vi "Target Main.vi"() -> ()   [LabVIEW 2014]
doc: "This application launches and executes the Tag Bus Data framework configuration for the specified target alias. This is a simple example of the framework API functions, but may also be a suitable starting point for a Host UI or Thick Client that is running a local version of the framework."
uses:
  <vilib>/NI/Module Execution Interface/Engine Runtime/Execution States.ctl
  <vilib>/NI/Module Execution Interface/Engine Runtime/Fault.ctl
  <vilib>/NI/Tag Bus Module Framework/runtime/error classification.ctl
  <vilib>/userdefined/High Color/nirio_resource_hc.ctl
  <vilib>/NI/Module Execution Interface/Engine Runtime/Engine Runtime Interface.lvclass
  <vilib>/NI/DCAF/Tag Editor Core/Framework Configuration Classes/target runtime/PL_Target Runtime.lvclass
  <vilib>/NI/Tag Bus Module Framework/FPGA manager/FPGA manager.lvlib
  <vilib>/rvi/interface/nirviOpenFPGA/nirviOpenFPGA.xnode
  <vilib>/NI/Tag Bus Module Framework/FPGA manager/methods.ctl
  <vilib>/NI/Tag Bus Module Framework/runtime/TBM module execution interface.lvclass
panel:
  in  "configuration file path":path=path "/home/lvuser/DCAFshm.pcfg"
  in  "target alias":string="cRIO"
  out "engine status":T4(array[cluster])
  out "stop":bool
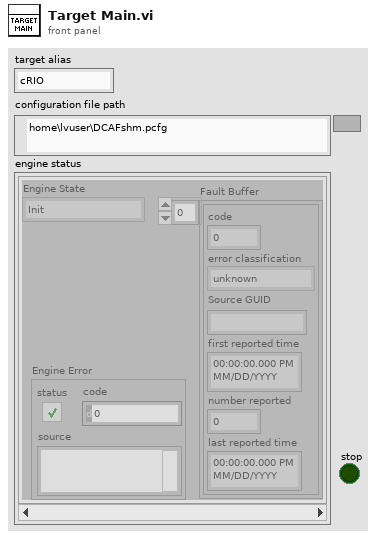
[diagram p1: front panel]
types:
  T1 = typedef "Engine Runtime Interface.lvclass/Execution States.ctl" = enum16{"Init", "Pre-Operational", "Safe-Operational", "Operational", "Stopped"}
  T2 = typedef "Engine Runtime Interface.lvclass/Fault.ctl" = cluster{"code":i32, "error classification":T3, "Source GUID":string, "first reported time":timestamp, "number reported":u32, "last reported time":timestamp}
  T3 = typedef "TBM module execution interface.lvclass/error classification.ctl" = enum16{"unknown", "none", "trivial", "recoverable", "critical"}
  T4 = cluster{"Engine State":T1, "Fault Buffer":T2[], "Engine Error":errorcluster}[]
  T5 = typedef "FPGA manager.lvlib/methods.ctl" = enum16{"initialize bitfile", "cache bitfile", "locate bitfile", "close bitfile", "clear manager"}
  T6 = typedef "nirio_resource_hc.ctl" = tag
  T7 = cluster{"Engine State":T1, "faults":T2[], "Engine Error":errorcluster}
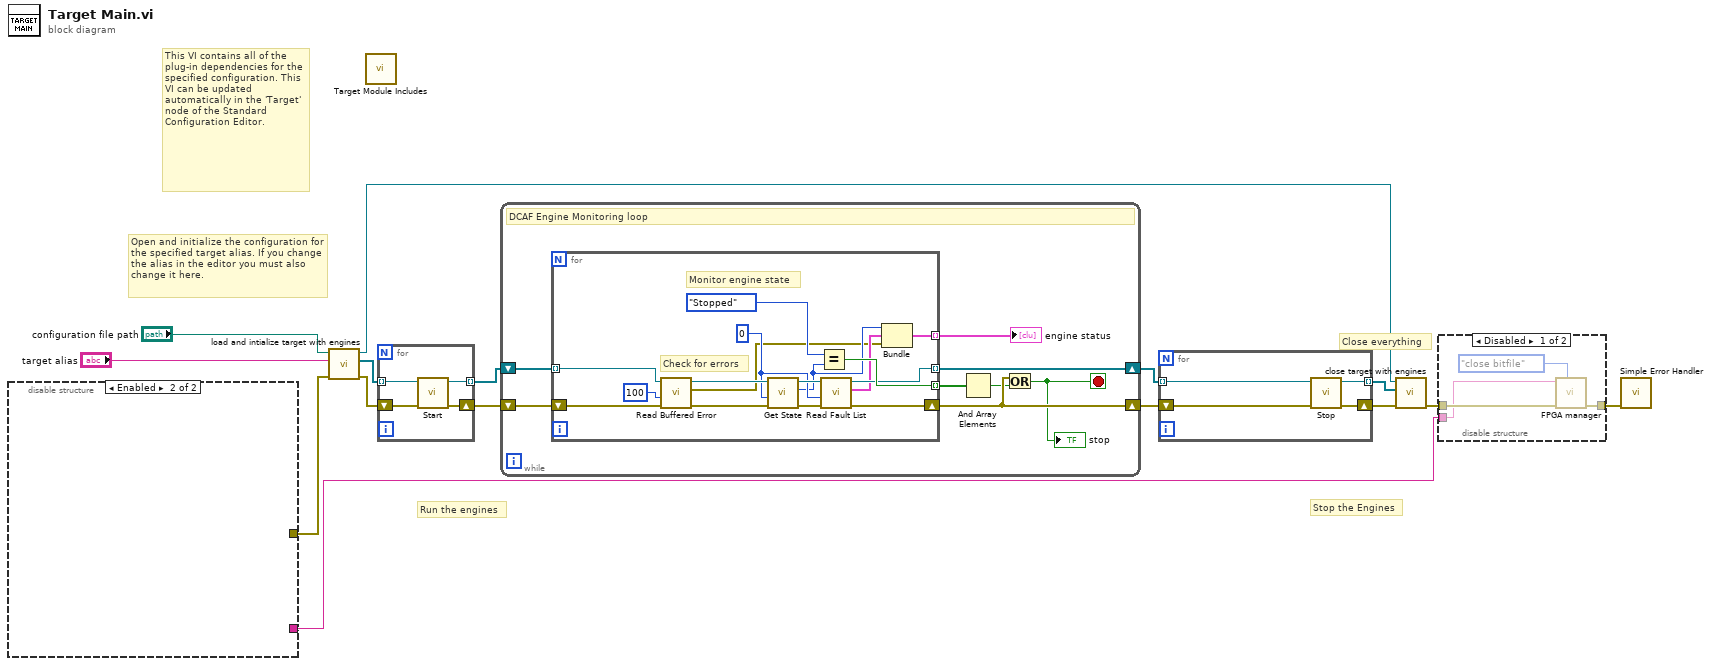
[diagram p0: block diagram]
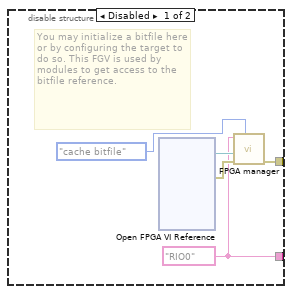
[diagram p3: hidden frame]
diagram:
  # "Open and initialize the configuration for the specified target alias. If you change the alias in the editor you must also change it here."
  # "Close everything"
  # "Stop the Engines"
  # "This VI contains all of the plug-in dependencies for the specified configuration. This VI can be updated automatically in the 'Target' node of the Standard Configuration Editor."
  # "Run the engines"
  n1 = disable-structure shown="Enabled" {
    disable-tunnel: [w20 _] -> w2
    disable-tunnel: [w16 _] -> w5
    frame Disabled {
      w16 = T6 "RIO0" ("RIO resource")
      # "You may initialize a bitfile here or by configuring the target to do so. This FGV is used by modules to get access to the bitfile reference."
      n2 = xnode "Open FPGA VI Reference"() -> ("FPGA VI Reference Out"=w18:refnum<k20>, "error out"=w19:errorcluster)  [unwired: 2 in]
      n3 = call <vilib>:"FPGA manager.vi"("action"=methods."cache bitfile", "error in"=w19, "bitfile to cache"=w18, "RIO resource"=w16) -> ("error out"=w20:errorcluster)  [unwired: 5 in, 2 out]
    }
    frame Enabled {
    }
  }
  n4 = call <vilib>:"load and intialize target with engines.vi"("error in"=w2, "target alias"="target alias", "file path"="configuration file path") -> ("error out"=w12:errorcluster, "engine runtime interfaces"=w11:refnum<class "Engine Runtime Interface.lvclass">[], "target runtime"=w8:refnum<class "PL_Target Runtime.lvclass">)  [unwired: 6 in]
  n5 = call "Target Module Includes.vi"() -> ()  [unwired: 12 in]
  n6 = for {
    tunnel: [w24] -> w15 mode=indexing
    tunnel: w11 -> [w21] mode=indexing
    shift-right: [w23] -> w4
    shift-left: w12 -> [w22]
    n7 = call-dynamic "Start.vi"("error in"=w22, "Engine Runtime Interface in"=w21) -> ("error out"=w23:errorcluster, "Engine Runtime Interface out"=w24:refnum<class "Engine Runtime Interface.lvclass">)  [unwired: 8 in]
  }
  n8 = while {
    shift-right: [w30] -> w14
    shift-left: w15 -> [w32]
    shift-right: [w29] -> w13
    shift-left: w4 -> [w31]
    stop <- w25 stop-if-true
    # "DCAF Engine Monitoring loop"
    n9 = for {
      tunnel: w32 -> [w48] mode=indexing
      tunnel: [w39] -> w30 mode=indexing
      tunnel: [w43] -> w27 mode=indexing
      shift-right: [w38] -> w29
      shift-left: w31 -> [w47]
      tunnel: [w33] -> w28 mode=indexing
      w37 = 0 ("timeout (-1)")
      # "Monitor engine state"
      # "Check for errors"
      n10 = call-dynamic "Read Buffered Error.vi"("error in"=w47, "timeout in ms (0)"=100, "Engine Runtime Interface in"=w48) -> ("error out"=w45:errorcluster, "Engine Error"=w34:errorcluster, "Engine Runtime Interface out"=w46:refnum<class "Engine Runtime Interface.lvclass">)  [unwired: 6 in]
      n11 = call-dynamic "Get State.vi"("error in"=w45, "timeout (-1)"=w37, "Engine Runtime Interface in"=w46) -> ("error out"=w41:errorcluster, "Engine State"=w36:T1, "Engine Runtime Interface out"=w40:refnum<class "Engine Runtime Interface.lvclass">)  [unwired: 6 in]
      n12 = Equal?(x=Execution_States."Stopped" ("Engine State"), y=w36) -> (x = y?=w43:bool)
      n13 = call-dynamic "Read Fault List.vi"("error in"=w41, "timeout (-1)"=w37, "Engine Runtime Interface in"=w40) -> ("error out"=w38:errorcluster, "faults"=w35:T2[], "Engine Runtime Interface out"=w39:refnum<class "Engine Runtime Interface.lvclass">)  [unwired: 6 in]
      n14 = Bundle("Engine State"=w36, "faults"=w35, "Engine Error"=w34) -> (w33:T7)  [unwired: 1 in]
    }
    "engine status" <- w28
    n15 = And Array Elements(Boolean array=w27) -> (logical AND=w26:bool)
    n16 = Or(x=w29, y=w26) -> (x .or. y?=w25:bool)
    "stop" <- w25
  }
  n17 = for {
    tunnel: w14 -> [w52] mode=indexing
    shift-right: [w49] -> w7
    shift-left: w13 -> [w51]
    tunnel: [w50] -> w9 mode=indexing
    n18 = call-dynamic "Stop.vi"("error in"=w51, "Engine Runtime Interface in"=w52) -> ("error out"=w49:errorcluster, "Engine Runtime Interface out"=w50:refnum<class "Engine Runtime Interface.lvclass">)  [unwired: 8 in]
  }
  n19 = call <vilib>:"close target with engines.vi"("error in"=w7, "Engine Runtime Interfaces"=w9, "Target Runtime"=w8) -> ("error out"=w3:errorcluster)  [unwired: 8 in]
  n20 = disable-structure shown="Disabled" {
    disable-tunnel: [w55 w57] -> w1
    disable-tunnel: w3 -> [w56 w57]
    disable-tunnel: w5 -> [w53 _]
    frame Disabled {
      n21 = call <vilib>:"FPGA manager.vi"("action"=methods."close bitfile", "error in"=w56, "RIO resource"=w53) -> ("error out"=w55:errorcluster)  [unwired: 6 in, 2 out]
    }
    frame Enabled {
    }
  }
  n22 = call <vilib>:"Simple Error Handler.vi"("error in (no error)"=w1) -> ()  [unwired: 4 in, 5 out]
